vi "Read Request.vi"(0 "connection ID":refnum<k5>, 11 "error in (no error)":errorcluster) -> (4 "connection ID out":refnum<k5>, 8 "TCPMessage":T1, 15 "error out":errorcluster)   [LabVIEW 2020, in "epl-network.lvlib"]
uses:
  epl-network.lvlib
  Typedefs/TCP Message.ctl
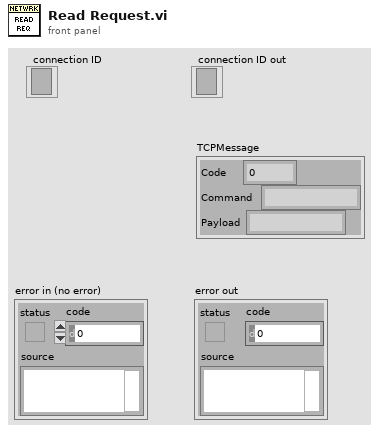
[diagram p1: front panel]
types:
  T1 = typedef "epl-network.lvlib/TCP Message.ctl" = cluster{"Code":i32, "Command":string, "Payload":string}
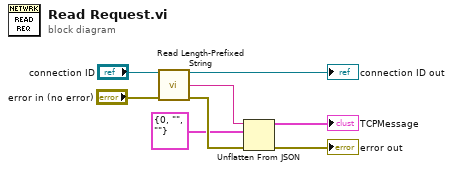
[diagram p0: block diagram]
diagram:
  n1 = call "Read Length-Prefixed String.vi"("connection ID"="connection ID", "error in (no error)"="error in (no error)") -> ("connection ID out"=→"connection ID out":refnum<k5>, "string"=w5:string, "error out"=w4:errorcluster)  [unwired: 11 in]
  n2 = Unflatten From JSON(JSON string=w5, type and defaults=T1 {"Code"=0, "Command"="", "Payload"=""} ("TcpMessage"), error in (no error)=w4) -> (value=→"TCPMessage":T1, error out=→"error out":errorcluster)  [unwired: 4 in]
